vi "Create Mask.vi"(0 "ToneCloud in":refnum<class "Tone Cloud.lvclass">, 7 "iRep":i32, 9 "iRow":i32, 11 "error in (no error)":errorcluster) -> (4 "ToneCloud out":refnum<class "Tone Cloud.lvclass">, 6 "row":cluster{"index":i32[], "level":dbl[]}, 8 "amplitudes":dbl[](array[numeric]), 10 "indices":i32[](array[numeric]), 15 "error out":errorcluster)   [LabVIEW 2015, in "Tone Cloud.lvclass"]
uses:
  Tone Cloud.lvclass
  Tone Cloud.lvclass/Tone Cloud.ctl
  Utility VIs/Math VIs/LinSpace (x0-dx-npts).vi
  Utility VIs/Math VIs/dB to Linear (scalar).vi
  <vilib>/Analysis/1siggen.llb/Riffle Array (I32).vi
  <vilib>/Analysis/NI_AALBase.lvlib
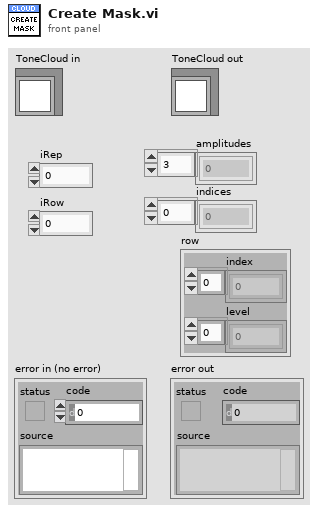
[diagram p1: front panel]
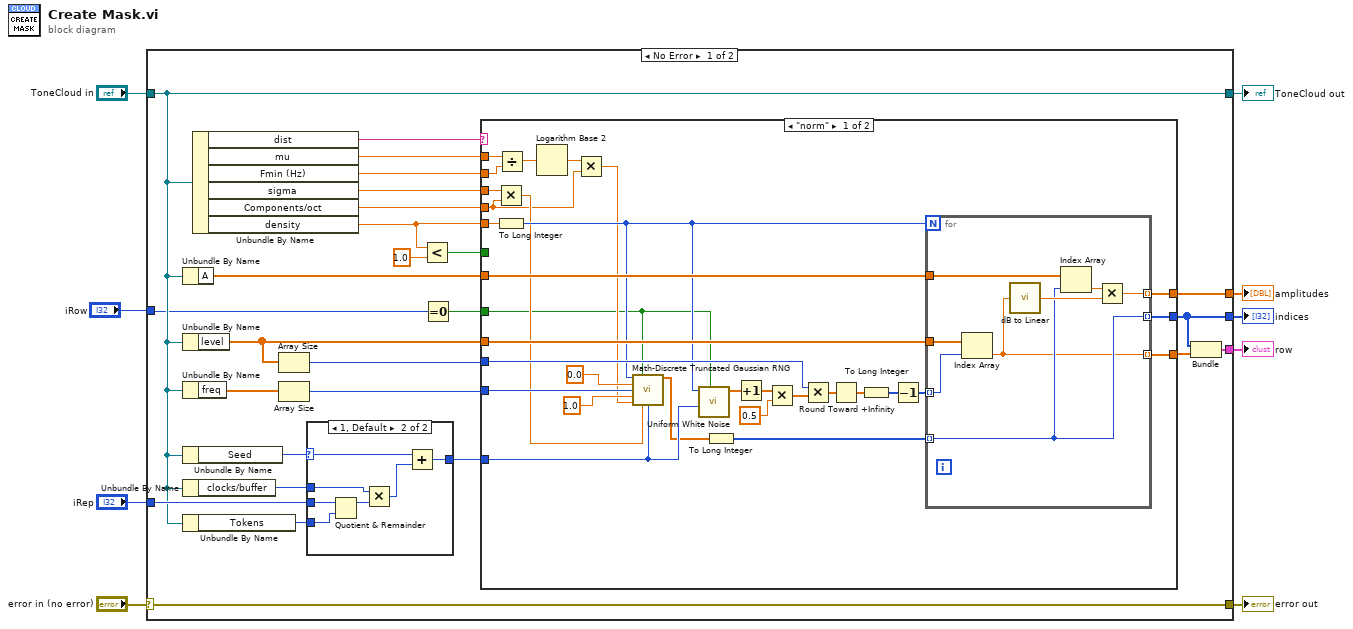
[diagram p0: block diagram]
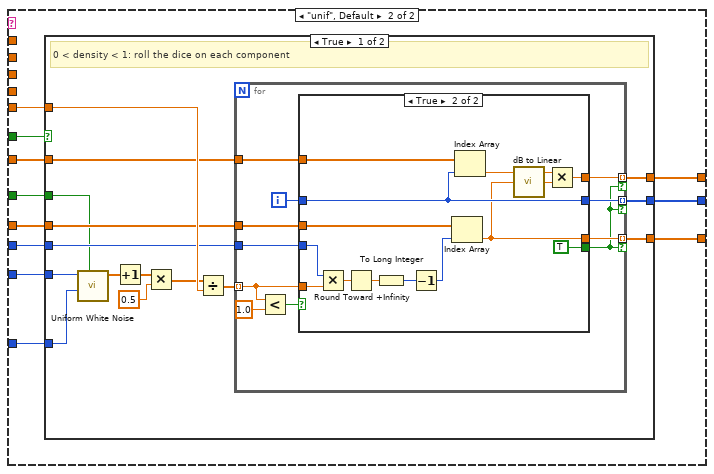
[diagram p2: hidden frame]
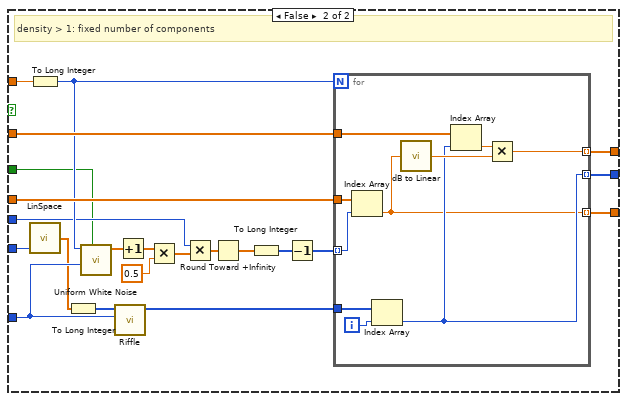
[diagram p4: hidden frame]
diagram:
  n1 = case shown="No Error" "error in (no error)" {
    selector: "error in (no error)" -> [w35 w166]
    tunnel: [w35 w166] -> w8
    tunnel: [w22 w165] -> w6
    tunnel: "ToneCloud in" -> [w22 w165]
    tunnel: "iRep" -> [w30 _]
    tunnel: [w24 _] -> w4
    tunnel: [w11 _] -> w3
    tunnel: "iRow" -> [w19 _]
    tunnel: [w10 _] -> w1
    frame No Error {
      n2 = Unbundle By Name(w22) -> ("A"=w25:dbl[])
      n3 = Unbundle By Name(w22) -> ("level"=w26:dbl[])
      n4 = Unbundle By Name(w22) -> ("freq"=w29:dbl[])
      n5 = Unbundle By Name(w22) -> ("Seed"=w31:i32)
      n6 = Unbundle By Name(w22) -> ("clocks/buffer"=w21:i32)
      n7 = Unbundle By Name(w22) -> ("Tokens"=w23:i32)
      n8 = Unbundle By Name(w22) -> ("dist"=w17:string, "mu"=w16:dbl, "Fmin (Hz)"=w13:dbl, "sigma"=w15:dbl, "Components/oct"=w14:dbl, "density"=w32:dbl)
      n9 = Array Size(array=w26) -> (size(s)=w27:i32)
      n10 = Array Size(array=w29) -> (size(s)=w28:i32)
      n11 = case shown="1, Default" w31 {
        selector: w31 -> [_ w161]
        tunnel: w30 -> [_ w164]
        tunnel: [_ w162] -> w20
        tunnel: w23 -> [_ w163]
        tunnel: w21 -> [_ w159]
        frame 0 {
        }
        frame 1, Default {
          n12 = Quotient & Remainder(x=w164, y=w163) -> (x-y*floor(x/y)=w160:i32)  [unwired: 1 out]
          n13 = Multiply(x=w159, y=w160) -> (x*y=w158:i32)
          n14 = Add(x=w161, y=w158) -> (x+y=w162:i32)
        }
      }
      n15 = Less?(x=w32, y=1.0) -> (x < y?=w33:bool)
      n16 = Equal To 0?(x=w19) -> (x = 0?=w18:bool)
      n17 = case shown="\"norm\"" w17 {
        tunnel: w33 -> [_ w85]
        tunnel: w32 -> [w66 w84]
        tunnel: w28 -> [w51 w83]
        tunnel: w27 -> [w63 w82]
        tunnel: w26 -> [w64 w81]
        tunnel: w25 -> [w65 w80]
        tunnel: [w55 w79] -> w24
        tunnel: [w38 w78] -> w11
        tunnel: w20 -> [w54 w77]
        tunnel: w18 -> [w39 w76]
        tunnel: w16 -> [w45 _]
        tunnel: w15 -> [w47 _]
        tunnel: w14 -> [w41 _]
        tunnel: w13 -> [w44 _]
        tunnel: [w37 w75] -> w12
        frame "norm" {
          n18 = Multiply(x=w47, y=w41) -> (x*y=w46:dbl)
          n19 = To Long Integer(number=w66) -> (32bit integer=w53:i32)
          n20 = Divide(x=w45, y=w44) -> (x/y=w43:dbl)
          n21 = Logarithm Base 2(1:w43) -> (0:w42:dbl)
          n22 = Multiply(x=w42, y=w41) -> (x*y=w40:dbl)
          n23 = call "Math-Discrete Truncated Gaussian RNG.vi"("samples"=w53, "reset"=w39, "Min"=0.0, "Max"=w51, "Step"=1.0, "mu"=w40, "sigma"=w46, "seed"=w54) -> ("Array"=w49:dbl[])  [unwired: 7 in]
          n24 = call <vilib>:"Uniform White Noise.vi"("initialize?"=w39, "seed"=w54, "samples"=w53) -> ("uniform white noise"=w62:dbl[])  [unwired: 7 in, 1 out]
          n25 = To Long Integer(number=w49) -> (32bit integer=w48:i32[])
          n26 = Increment(x=w62) -> (x+1=w61:dbl[])
          n27 = Multiply(x=w61, y=0.5) -> (x*y=w57:dbl[])
          n28 = Multiply(x=w63, y=w57) -> (x*y=w58:dbl[])
          n29 = Round Toward +Infinity(x=w58) -> (ceil(x): smallest int >= x=w59:dbl[])
          n30 = To Long Integer(number=w59) -> (32bit integer=w56:i32[])
          n31 = Decrement(x=w56) -> (x-1=w36:i32[])
          n32 = for {
            N: w53 -> [_]
            tunnel: w64 -> [w74]
            tunnel: w65 -> [w73]
            tunnel: [w72] -> w55 mode=indexing
            tunnel: [w68] -> w38 mode=indexing
            tunnel: w36 -> [w69] mode=indexing
            tunnel: w48 -> [w68] mode=indexing
            tunnel: [w67] -> w37 mode=indexing
            n33 = Index Array(array=w74, index=w69) -> (element=w67:dbl)
            n34 = call-poly "dB to Linear.vi"("dB"=w67) -> ("linear"=w70:dbl)
            n35 = Index Array(array=w73, index=w68) -> (element=w71:dbl)
            n36 = Multiply(x=w71, y=w70) -> (x*y=w72:dbl)
          }
        }
        frame "unif", Default {
          n37 = case shown="True" w85 {
            tunnel: w84 -> [w96 w140]
            tunnel: w77 -> [w100 w139]
            tunnel: w83 -> [w99 w138]
            tunnel: w82 -> [w95 w130]
            tunnel: w81 -> [w94 w146]
            tunnel: w80 -> [w93 w145]
            tunnel: [w92 w144] -> w79
            tunnel: [w91 w143] -> w78
            tunnel: w76 -> [w87 w128]
            tunnel: [w86 w127] -> w75
            frame True {
              # "0 < density < 1: roll the dice on each component"
              n38 = call <vilib>:"Uniform White Noise.vi"("initialize?"=w87, "seed"=w100, "samples"=w99) -> ("uniform white noise"=w98:dbl[])  [unwired: 7 in, 1 out]
              n39 = Increment(x=w98) -> (x+1=w90:dbl[])
              n40 = Multiply(x=w90, y=0.5) -> (x*y=w89:dbl[])
              n41 = Divide(x=w89, y=w96) -> (x/y=w97:dbl[])
              n42 = for {
                tunnel: w97 -> [w111] mode=indexing
                tunnel: w95 -> [w109]
                tunnel: w94 -> [w108]
                tunnel: w93 -> [w106]
                tunnel: [w105] -> w92 mode=indexing if=w101
                tunnel: [w103] -> w91 mode=indexing if=w101
                tunnel: [w102] -> w86 mode=indexing if=w101
                i -> [w104]
                n43 = Less?(x=w111, y=1.0) -> (x < y?=w107:bool)
                n44 = case shown="True" w107 {
                  tunnel: w111 -> [_ w114]
                  tunnel: w109 -> [_ w125]
                  tunnel: w108 -> [_ w122]
                  tunnel: w106 -> [_ w120]
                  tunnel: [_ w118] -> w105
                  tunnel: w104 -> [_ w116]
                  tunnel: [_ w116] -> w103
                  tunnel: [_ TRUE] -> w101
                  tunnel: [_ w113] -> w102
                  frame False {
                  }
                  frame True {
                    n45 = Multiply(x=w125, y=w114) -> (x*y=w124:dbl)
                    n46 = Round Toward +Infinity(x=w124) -> (ceil(x): smallest int >= x=w123:dbl)
                    n47 = To Long Integer(number=w123) -> (32bit integer=w121:i32)
                    n48 = Decrement(x=w121) -> (x-1=w112:i32)
                    n49 = Index Array(array=w122, index=w112) -> (element=w113:dbl)
                    n50 = Index Array(array=w120, index=w116) -> (element=w119:dbl)
                    n51 = call-poly "dB to Linear.vi"("dB"=w113) -> ("linear"=w117:dbl)
                    n52 = Multiply(x=w119, y=w117) -> (x*y=w118:dbl)
                  }
                }
              }
            }
            frame False {
              # "density > 1: fixed number of components"
              n53 = To Long Integer(number=w140) -> (32bit integer=w134:i32)
              n54 = call-poly "LinSpace.vi"("npts"=w138) -> ("Array"=w137:dbl[])  [unwired: 3 in, 1 out]
              n55 = To Long Integer(number=w137) -> (32bit integer=w136:i32[])
              n56 = call <vilib>:"Uniform White Noise.vi"("initialize?"=w128, "seed"=w139, "samples"=w134) -> ("uniform white noise"=w147:dbl[])  [unwired: 7 in, 1 out]
              n57 = call-poly <vilib>:"Riffle.vi"("seed"=w139, "X"=w136) -> ("Riffled {X}"=w135:i32[])  [unwired: 7 in, 2 out]
              n58 = Increment(x=w147) -> (x+1=w142:dbl[])
              n59 = Multiply(x=w142, y=0.5) -> (x*y=w131:dbl[])
              n60 = Multiply(x=w130, y=w131) -> (x*y=w132:dbl[])
              n61 = Round Toward +Infinity(x=w132) -> (ceil(x): smallest int >= x=w133:dbl[])
              n62 = To Long Integer(number=w133) -> (32bit integer=w129:i32[])
              n63 = Decrement(x=w129) -> (x-1=w126:i32[])
              n64 = for {
                N: w134 -> [_]
                tunnel: w146 -> [w157]
                tunnel: w145 -> [w156]
                tunnel: [w155] -> w144 mode=indexing
                tunnel: [w149] -> w143 mode=indexing
                tunnel: w135 -> [w151]
                tunnel: w126 -> [w152] mode=indexing
                tunnel: [w148] -> w127 mode=indexing
                i -> [w150]
                n65 = Index Array(array=w157, index=w152) -> (element=w148:dbl)
                n66 = Index Array(array=w151, index=w150) -> (element=w149:i32)
                n67 = call-poly "dB to Linear.vi"("dB"=w148) -> ("linear"=w153:dbl)
                n68 = Index Array(array=w156, index=w149) -> (element=w154:dbl)
                n69 = Multiply(x=w154, y=w153) -> (x*y=w155:dbl)
              }
            }
          }
        }
      }
      n70 = Bundle(w11, w12) -> (w10:cluster{i32[], dbl[]})  [unwired: 1 in]
    }
    frame Error {
    }
  }
  "error out" <- w8
  "ToneCloud out" <- w6
  "indices" <- w3
  "amplitudes" <- w4
  "row" <- w1
